vi "Initialize_filesystemd_events_registration_and_queue.vi"(8 "error in (no error)":errorcluster, 11 "Settings":T1={"SourceDirectory"=path "", "Save"=enum."off", "Timeout"={"Value"=0.0, "Min"=0.0, "Max"=0.0, "StepSize"=0.0, "Tolerance"=0.0, "valueactual"=0.0}, "CleanSource"=enum."off", "NumFiles"={"Value"=0.0, "Min"=0.0, "Max"=0.0, "StepSize"=0.0, "Tolerance"=0.0, "valueactual"=0.0}, "FileSearchPattern"="", "MaxAllowedDirFiles"={"Value"=0.0, "Min"=0.0, "Max"=0.0, "StepSize"=0.0, "Tolerance"=0.0, "valueactual"=0.0}, "localsavingpath"=path "", "FileMoveDelay"={"Value"=100.0, "Min"=-1.0, "Max"=100000.0, "StepSize"=1.0, "Tolerance"=0.0, "valueactual"=0.0}}) -> (0 "error out":errorcluster, 1 "event callback refnum":refnum<k27>, 2 "file system watcher reference":refnum<k24>, 3 "Queue out":refnum<queue>)   [LabVIEW 2020, in "FileCopyEventBased.lvclass"]
uses:
  FileCopyEventBased.lvclass
  SettingsTypdef.ctl
  OnOffTypeDef.ctl
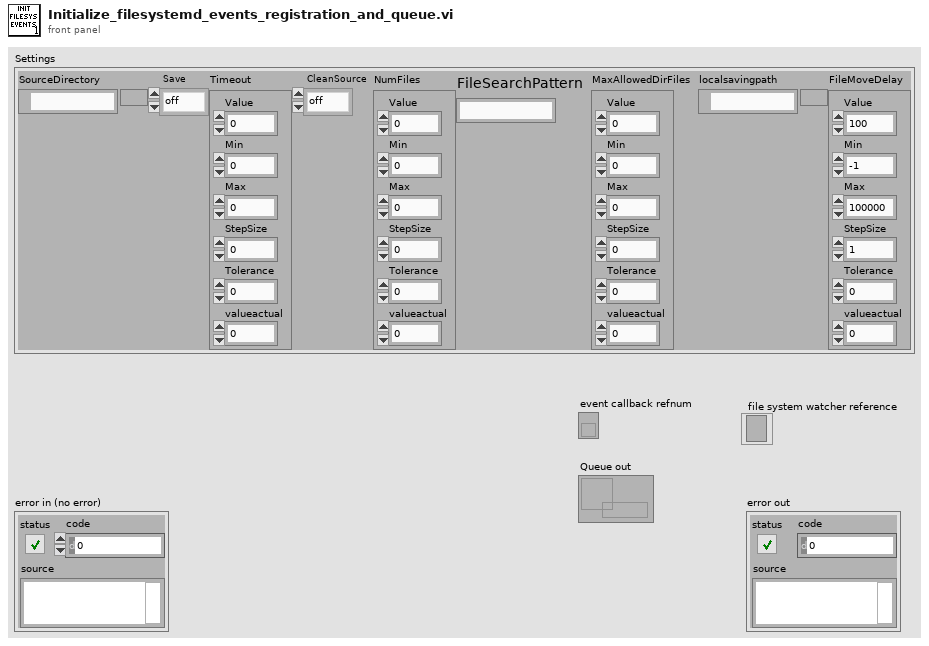
[diagram p1: front panel]
types:
  T1 = typedef "FileCopyEventBased.lvclass/SettingsTypdef.ctl" = cluster{"SourceDirectory":path, "Save":T2, "Timeout":cluster{"Value":dbl, "Min":dbl, "Max":dbl, "StepSize":dbl, "Tolerance":dbl, "valueactual":dbl}, "CleanSource":T2, "NumFiles":cluster{"Value":dbl, "Min":dbl, "Max":dbl, "StepSize":dbl, "Tolerance":dbl, "valueactual":dbl}, "FileSearchPattern":string, "MaxAllowedDirFiles":cluster{"Value":dbl, "Min":dbl, "Max":dbl, "StepSize":dbl, "Tolerance":dbl, "valueactual":dbl}, "localsavingpath":path, "FileMoveDelay":cluster{"Value":dbl, "Min":dbl, "Max":dbl, "StepSize":dbl, "Tolerance":dbl, "valueactual":dbl}}
  T2 = typedef "OnOffTypeDef.ctl" = enum16{"off", "on"}
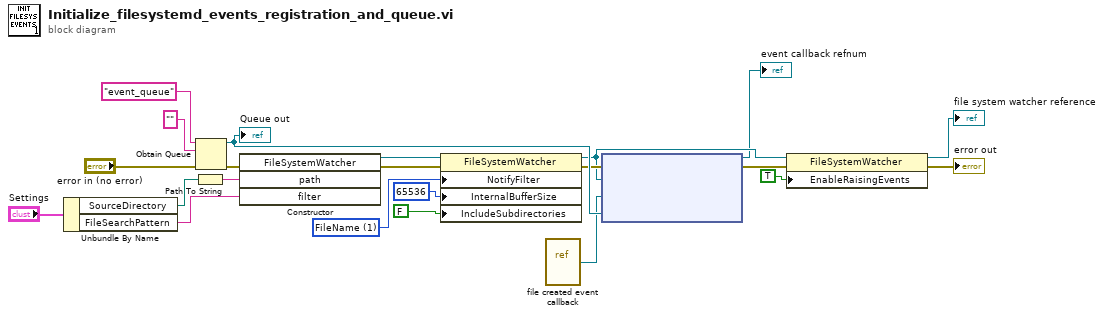
[diagram p0: block diagram]
diagram:
  w8 = 1 items=["FileName"=1, "DirectoryName"=2, "Attributes"=4, "Size"=8, "LastWrite"=16, "LastAccess"=32, "CreationTime"=64, "Security"=256] ("NotifyFilter")
  n1 = Unbundle By Name("Settings") -> ("SourceDirectory"=w16:path, "FileSearchPattern"=w18:string)
  n2 = Path To String(path=w16) -> (string=w17:string)
  n3 = Obtain Queue(name (unnamed)="event_queue", element data type="", error in (no error)="error in (no error)") -> (queue out=w20:refnum<queue>, error out=w12:errorcluster)  [unwired: 2 in, 1 out]
  "Queue out" <- w20
  n4 = constructor class="FileSystemWatcher"(error in=w12, "path"=w17, "filter"=w18) -> (reference out=w4:refnum<k24>, error out=w5:errorcluster)  [unwired: 2 in, 3 out]
  n5 = property class="FileSystemWatcher"(reference=w4, error in=w5, "NotifyFilter"=w8, "InternalBufferSize"=65536, "IncludeSubdirectories"=FALSE) -> (reference out=w11:refnum<k24>, error out=w15:errorcluster)
  n6 = vi-ref "file created event callback.vi"() -> ("vi reference"=w13:refnum<vi>)
  n7 = node(w15, w11, w13, w20) -> (→"event callback refnum":refnum<k27>, w9:errorcluster)  [unwired: 1 in]
  n8 = property class="FileSystemWatcher"(reference=w11, error in=w9, "EnableRaisingEvents"=TRUE) -> (reference out=→"file system watcher reference":refnum<k24>, error out=→"error out":errorcluster)
